vi "Init.vi"(8 "error in (no error)":errorcluster, 11 "Data":variant) -> (0 "error out":errorcluster)   [LabVIEW 2018, in "RT - Analysis.lvlib"]
doc: "This subVI enqueues the named action in to the communications queue along with the input data."
uses:
  RT - Analysis.lvlib
  Private Controls/Module Data.ctl
  Private Controls/Module Action.ctl
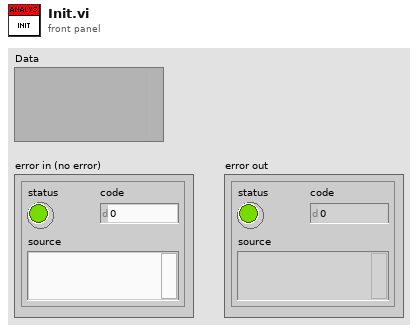
[diagram p1: front panel]
types:
  T1 = typedef "RT - Analysis.lvlib/Module Data.ctl" = cluster{"Data":variant, "Action":T2}
  T2 = typedef "RT - Analysis.lvlib/Module Action.ctl" = enum16{"Raw Data", "Set Repair Level", "APU Setup Info", "Init", "Error", "Set Highpass", "Set Accel Sens"}
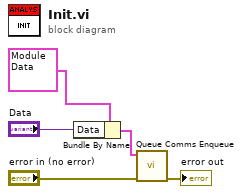
[diagram p0: block diagram]
diagram:
  n1 = Bundle By Name(cluster=T1 {"Data"=variant, "Action"=enum."Init"} ("element"), "Data"="Data") -> (w4:T1)
  n2 = call "Queue Comms Enqueue.vi"("error in (no error)"="error in (no error)", "element"=w4) -> ("error out"=→"error out":errorcluster)  [unwired: 9 in]
